vi "Front or Flank.vi"(10 "Enemy Direction":i32, 11 "Direction":i32) -> (3 "Front?":bool)   [LabVIEW 2014, in "Formics.lvclass"]
uses:
  Formics.lvclass
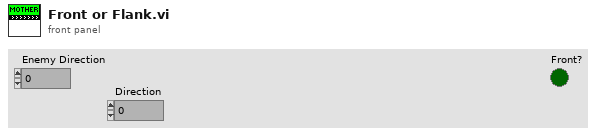
[diagram p1: front panel]
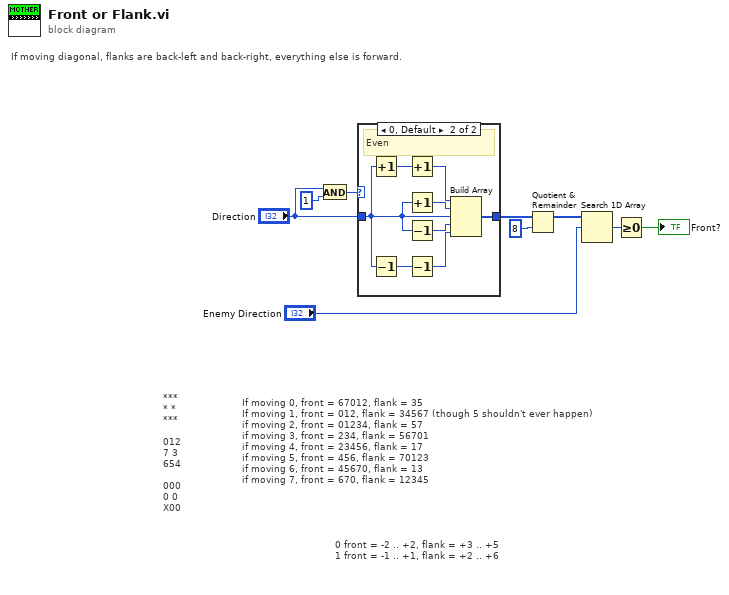
[diagram p0: block diagram]
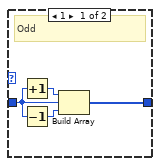
[diagram p2: hidden frame]
diagram:
  # "If moving diagonal, flanks are back-left and back-right, everything else is forward."
  # "***\n* *\n***\n\n012\n7 3\n654\n\n000\n0 0\nX00"
  # "0 front = -2 .. +2, flank = +3 .. +5\n1 front = -1 .. +1, flank = +2 .. +6"
  # "If moving 0, front = 67012, flank = 35\nIf moving 1, front = 012, flank = 34567 (though 5 shouldn't ever happen)\nif moving 2, front = 01234, flank = 57\nif moving 3, front = 234, flank = 56701\nif moving 4, front = 23456, flank = 17\nif moving 5, front = 456, flank = 70123\nif moving 6, front = 45670, flank = 13\nif moving 7, front = 670, flank = 12345"
  n1 = And(x="Direction", y=1) -> (x .and. y?=w8:i32)
  n2 = case shown="0, Default" w8 {
    tunnel: [w12 w19] -> w7
    tunnel: "Direction" -> [w10 w14]
    frame 1 {
      # "Odd"
      n3 = Increment(x=w10) -> (x+1=w13:i32)
      n4 = Decrement(x=w10) -> (x-1=w11:i32)
      n5 = Build Array(w13, w10, w11) -> (w12:i32[])
    }
    frame 0, Default {
      # "Even"
      n6 = Increment(x=w14) -> (x+1=w18:i32)
      n7 = Decrement(x=w14) -> (x-1=w16:i32)
      n8 = Increment(x=w18) -> (x+1=w21:i32)
      n9 = Increment(x=w14) -> (x+1=w20:i32)
      n10 = Decrement(x=w14) -> (x-1=w17:i32)
      n11 = Decrement(x=w16) -> (x-1=w15:i32)
      n12 = Build Array(w21, w20, w14, w17, w15) -> (w19:i32[])
    }
  }
  n13 = Quotient & Remainder(x=w7, y=8) -> (x-y*floor(x/y)=w4:i32[])  [unwired: 1 out]
  n14 = Search 1D Array(1D array=w4, element="Enemy Direction") -> (index of element=w2:i32)  [unwired: 1 in]
  n15 = Greater Or Equal To 0?(x=w2) -> (x >= 0?=→"Front?":bool)
